vi "DDS - Sin Syn.vi"(7 "Reset Accumulator":bool, 10 "Accumulator Increment":fxp<+,32,32>) -> (1 "Accumulator Value":fxp<+,32,32>, 2 "data out":i16 caption="Sine Data Out")   [LabVIEW 2015]
uses:
  <vilib>/rvi/FXPMathLib/FxpAdd/XNode/nifxpmath_Add.xnode
  <vilib>/rvi/FXPMathLib/sim/FxpSim.dll
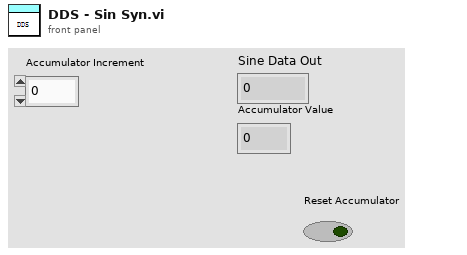
[diagram p1: front panel]
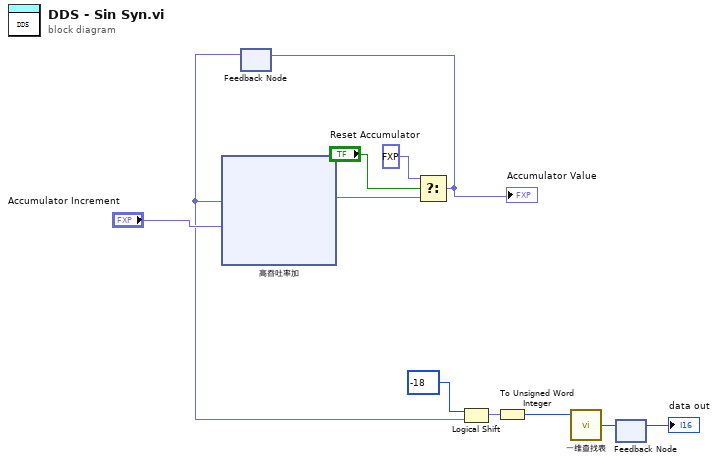
[diagram p0: block diagram]
diagram:
  n1 = feedback #1() -> (w2:fxp<+,32,32>)  [unwired: 1 in]
  n2 = xnode ("高吞吐率加")("x"=w2, "y"="Accumulator Increment") -> ("x+y"=w9:fxp<+,32,32>)
  n3 = Select(t=fxp<+,32,32> 0.0, s="Reset Accumulator", f=w9) -> (s? t:f=w10:fxp<+,32,32>)
  "Accumulator Value" <- w10
  n4 = feedback-in #1(w10) -> ()
  n5 = Logical Shift(y=i16 -18, x=w2) -> (x << y=w4:fxp<+,32,32>)
  n6 = To Unsigned Word Integer(number=w4) -> (unsigned 16bit integer=w3:u16)
  n7 = call "一维查找表"("address"=w3) -> ("data out"=w6:i16)  [unwired: 8 in]
  n8 = feedback-in #2(w6) -> ()
  n9 = feedback #2 ("反馈节点")() -> (→"data out":i16)  [unwired: 1 in]
